vi "Receive.vi"(8 "error in (no error)":errorcluster, 11 "SM1000-control in":refnum<class "HC-SM1000.lvclass">) -> (0 "error out":errorcluster, 2 "Return string":string, 3 "SM1000-control out":refnum<class "HC-SM1000.lvclass">)   [LabVIEW 2013, in "HardwareCharacterization.lvlib" / "HC-SM1000.lvclass"]
uses:
  HC-SM1000.lvclass
  HC-SM1000.lvclass/HC-SM1000.ctl
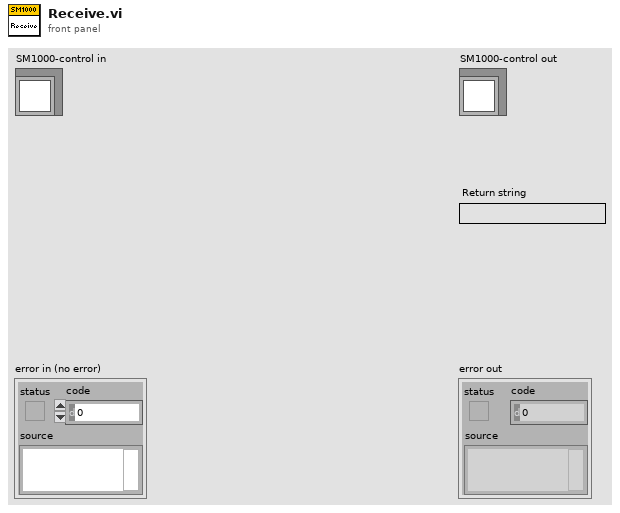
[diagram p1: front panel]
types:
  T1 = enum16{"Standard", "Buffered", "CRLF", "Immediate"}
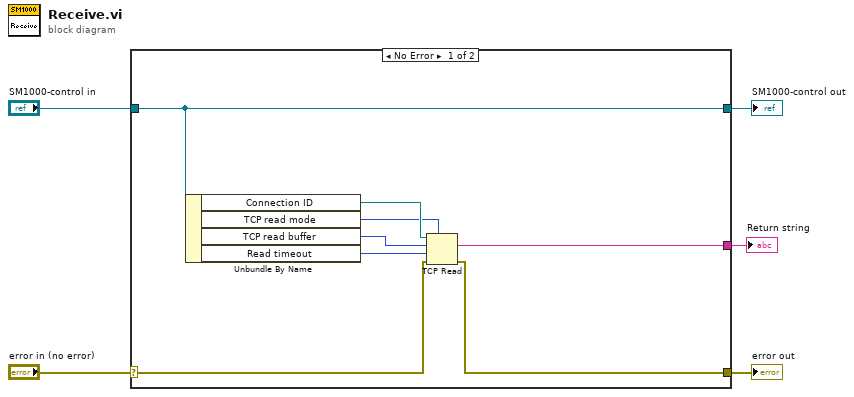
[diagram p0: block diagram]
diagram:
  n1 = case shown="No Error" "error in (no error)" {
    selector: "error in (no error)" -> [w10 w15]
    tunnel: [w9 w15] -> w4
    tunnel: [w13 w14] -> w2
    tunnel: "SM1000-control in" -> [w13 w14]
    tunnel: [w8 _] -> w1
    frame No Error {
      n2 = Unbundle By Name(w13) -> ("Connection ID"=w12:refnum<k5>, "TCP read mode"=w7:T1, "TCP read buffer"=w6:i32, "Read timeout"=w11:i32)
      n3 = TCP Read(connection ID=w12, bytes to read=w6, error in (no error)=w10, 7:w7, 9:w11) -> (data out=w8:string, error out=w9:errorcluster)  [unwired: 1 out]
    }
    frame Error {
    }
  }
  "error out" <- w4
  "SM1000-control out" <- w2
  "Return string" <- w1
